vi "Motor controller.vi"   [LabVIEW 2012]
uses:
  Motors Values.vi
  BotStatus.vi
types:
  T1 = typedef "WPI_ServoDeviceRef.ctl" = cluster{"DeviceStatus":errorcluster, "Digital Module":T2, "PWM Channel":T3, "DeadBand":T4}
  T2 = typedef "FPGA_TypedefDigitalModule.ctl" = enum16{"Digital Module 1", "Digital Module 2"}
  T3 = typedef "FPGA_DIOPWMChannel.ctl" = enum8{"PWM 1", "PWM 2", "PWM 3", "PWM 4", "PWM 5", "PWM 6", "PWM 7", "PWM 8", "PWM 9", "PWM 10", "Invalid"}
  T4 = typedef "WPI_PWMDeadband.ctl" = cluster{"Name":string, "maxPositivePwm":i32, "minPositivePwm":i32, "centerPwm":i32, "maxNegativePwm":i32, "minNegativePwm":i32, "angularRange":u16}
  T5 = typedef "WPI_MotorControlDeviceRef.ctl" = cluster{"DeviceStatus":errorcluster, "Type":enum16{"PWM", "CAN"}, "PWM":cluster{"Digital Module":T2, "PWM Channel":T3, "DeadBand":T4}, "CAN":cluster{"Device Number":u8, "Control Mode":T6, "Semaphore":T7, "Max Vout":dbl}, "Invert":bool, "TransformRef":T8, "InvTransformRef":T8}
  T6 = typedef "WPI_CANJaguar_ControlMode.ctl" = enum8{"Percent VBus", "Current", "Speed", "Position", "Voltage"}
  T7 = typedef "Semaphore RefNum" = refnum<k1>
  T8 = typedef "WPI_PWMTransform_ConPane.ctl" = refnum<vi>
  T9 = typedef "WPI_RelayDevRef.ctl" = cluster{"DevStatus":errorcluster, "Relay Channel":T10, "Digital Module":T2, "Relay Direction":T11}
  T10 = typedef "FPGA_DIORelayChannel.ctl" = enum8{"Relay 1", "Relay 2", "Relay 3", "Relay 4", "Relay 5", "Relay 6", "Relay 7", "Relay 8", "Invalid"}
  T11 = typedef "WPI_RelayDirection.ctl" = enum16{"Both directions", "Forward only", "Reverse only"}
  T12 = typedef "WPI_RelayValue.ctl" = enum16{"Off", "On", "Forward", "Reverse"}
  T13 = typedef "WPI_DigitalInputDevRef.ctl" = cluster{"DevStatus":errorcluster, "DIO Channel":T14, "Digital Module":T2}
  T14 = typedef "FPGA_DIOChannel.ctl" = enum8{"DIO 1", "DIO 2", "DIO 3", "DIO 4", "DIO 5", "DIO 6", "DIO 7", "DIO 8", "DIO 9", "DIO 10", "DIO 11", "DIO 12", "DIO 13", "DIO 14", "Invalid"}
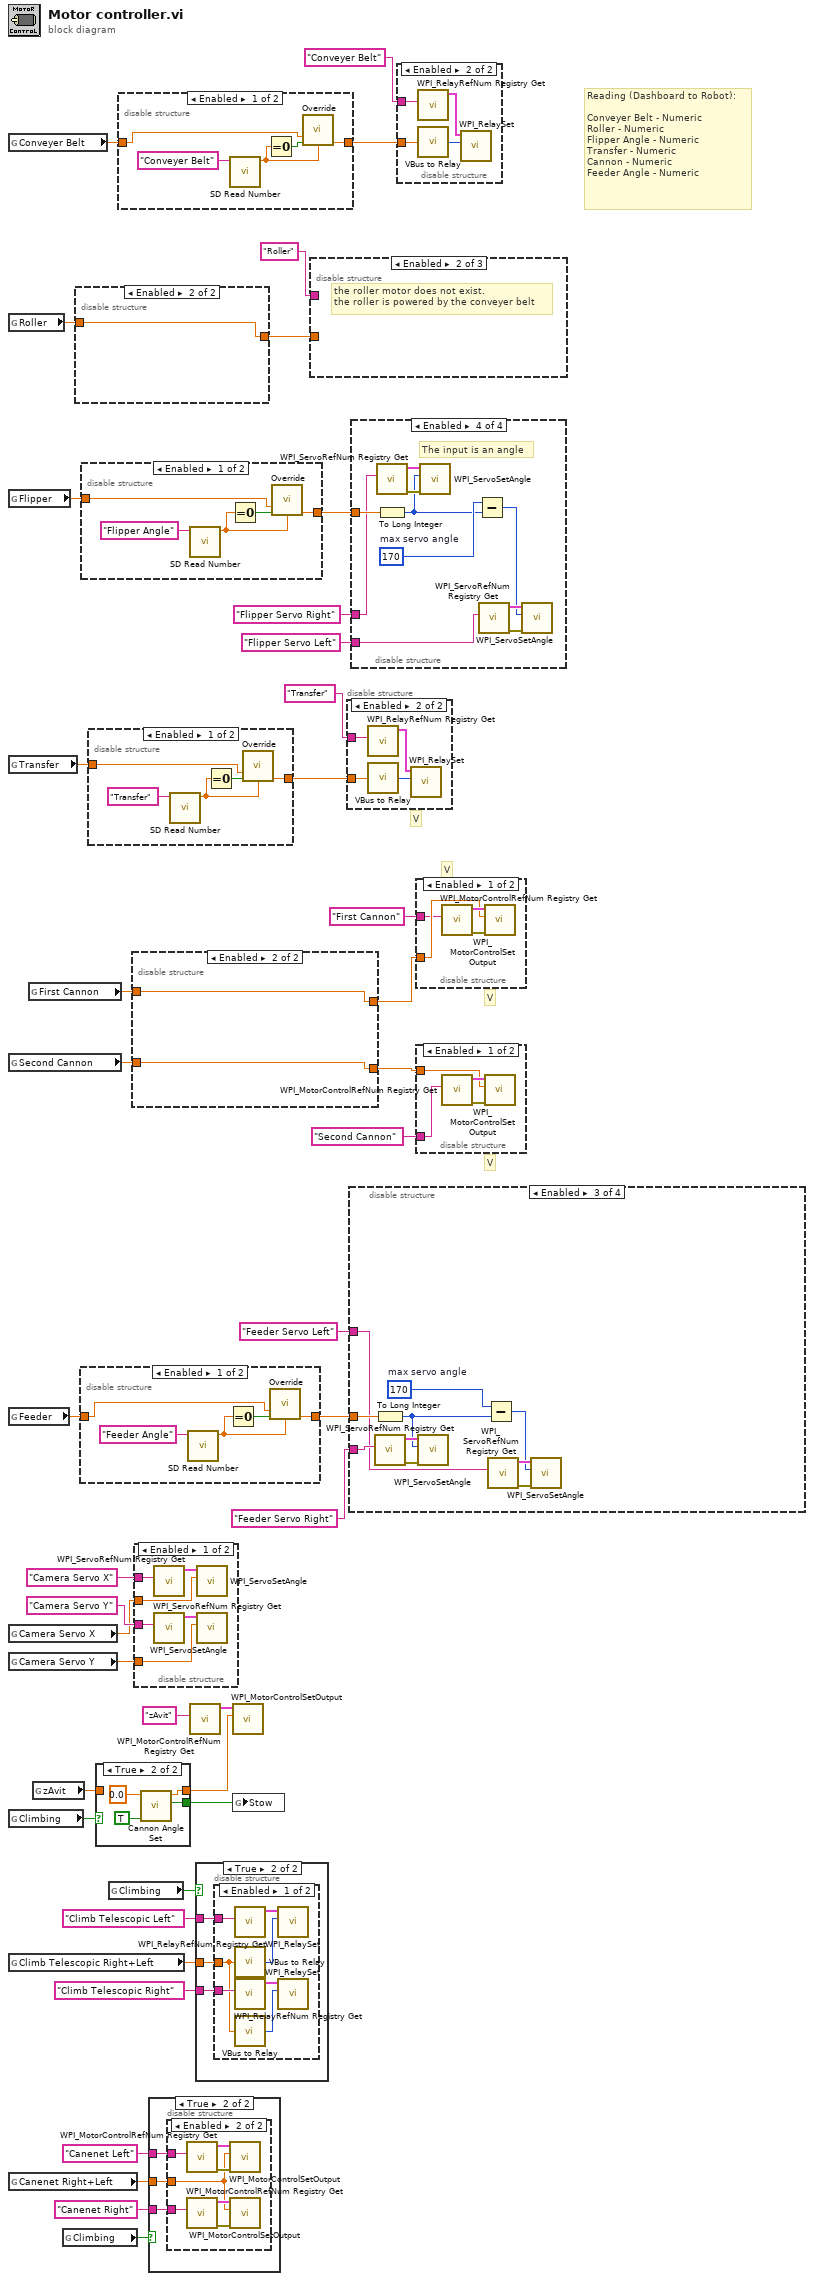
[diagram p0: block diagram]
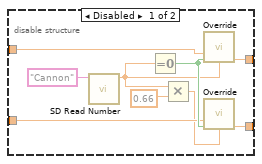
[diagram p3: hidden frame]
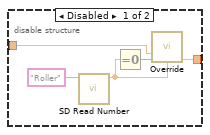
[diagram p6: hidden frame]
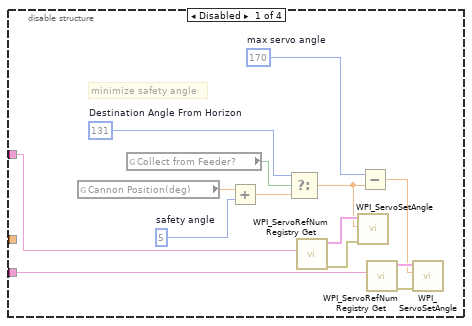
[diagram p9: hidden frame]
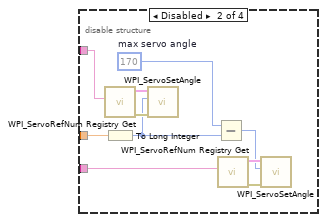
[diagram p10: hidden frame]
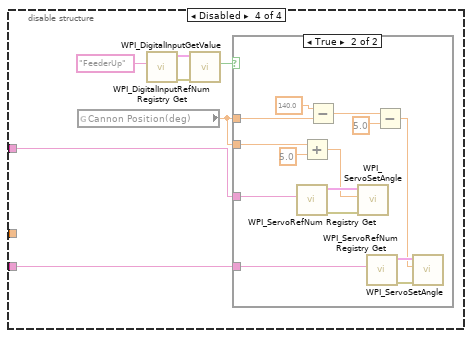
[diagram p11: hidden frame]
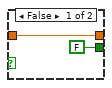
[diagram p13: hidden frame]
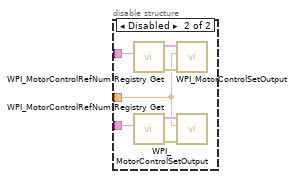
[diagram p17: hidden frame]
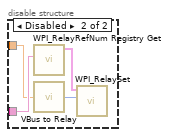
[diagram p18: hidden frame]
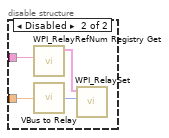
[diagram p19: hidden frame]
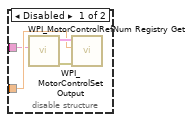
[diagram p20: hidden frame]
diagram:
  # "Reading (Dashboard to Robot):\n\nConveyer Belt - Numeric\nRoller - Numeric\nFlipper Angle - Numeric\nTransfer - Numeric\nCannon - Numeric\nFeeder Angle - Numeric"
  # "V"
  # "V"
  # "V"
  # "V"
  n1 = global read "Motors Values.vi" "Conveyer Belt"() -> (w13:dbl)
  n2 = global read "Motors Values.vi" "Roller"() -> (w12:dbl)
  n3 = global read "Motors Values.vi" "Flipper"() -> (w10:dbl)
  n4 = global read "Motors Values.vi" "Transfer"() -> (w8:dbl)
  n5 = global read "Motors Values.vi" "Second Cannon"() -> (w4:dbl)
  n6 = global read "Motors Values.vi" "Feeder"() -> (w1:dbl)
  n7 = global read "Motors Values.vi" "Camera Servo X"() -> (w16:dbl)
  n8 = global read "Motors Values.vi" "Camera Servo Y"() -> (w15:dbl)
  n9 = global read "BotStatus.vi" "Climbing"() -> (w25:bool)
  n10 = global read "Motors Values.vi" "Climb Telescopic Right+Left"() -> (w33:dbl)
  n11 = global read "Motors Values.vi" "Canenet Right+Left"() -> (w26:dbl)
  n12 = global read "Motors Values.vi" "First Cannon"() -> (w6:dbl)
  n13 = global read "Motors Values.vi" "zAvit"() -> (w24:dbl)
  n14 = global read "BotStatus.vi" "Climbing"() -> (w27:bool)
  n15 = disable-structure shown="Enabled" {
    disable-tunnel: w12 -> [w43 w47]
    disable-tunnel: [w42 w47] -> w11
    frame Disabled {
      n16 = call <vilib>:"SD Read Number.vi"("Name"="Roller") -> ("Numeric"=w45:dbl)  [unwired: 8 in, 2 out]
      n17 = Equal To 0?(x=w45) -> (x = 0?=w46:bool)
      n18 = call "Override.vi"("Regualer"=w43, "Override"=w46, "Overriden"=w45) -> ("Output"=w42:dbl)  [unwired: 12 in]
    }
    frame Enabled {
    }
  }
  n19 = disable-structure shown="Enabled" {
    disable-tunnel: [w49 w53] -> w2
    disable-tunnel: w1 -> [w48 w53]
    frame Enabled {
      n20 = call <vilib>:"SD Read Number.vi"("Name"="Feeder Angle") -> ("Numeric"=w52:dbl)  [unwired: 8 in, 2 out]
      n21 = Equal To 0?(x=w52) -> (x = 0?=w51:bool)
      n22 = call "Override.vi"("Regualer"=w48, "Override"=w51, "Overriden"=w52) -> ("Output"=w49:dbl)  [unwired: 12 in]
    }
    frame Disabled {
    }
  }
  n23 = disable-structure shown="Enabled" {
    disable-tunnel: w10 -> [w55 w59]
    disable-tunnel: [w54 w59] -> w9
    frame Enabled {
      n24 = call <vilib>:"SD Read Number.vi"("Name"="Flipper Angle") -> ("Numeric"=w57:dbl)  [unwired: 8 in, 2 out]
      n25 = Equal To 0?(x=w57) -> (x = 0?=w56:bool)
      n26 = call "Override.vi"("Regualer"=w55, "Override"=w56, "Overriden"=w57) -> ("Output"=w54:dbl)  [unwired: 12 in]
    }
    frame Disabled {
    }
  }
  n27 = disable-structure shown="Enabled" {
    disable-tunnel: w8 -> [w61 w65]
    disable-tunnel: [w60 w65] -> w7
    frame Enabled {
      n28 = call <vilib>:"SD Read Number.vi"("Name"="Transfer") -> ("Numeric"=w63:dbl)  [unwired: 8 in, 2 out]
      n29 = Equal To 0?(x=w63) -> (x = 0?=w62:bool)
      n30 = call "Override.vi"("Regualer"=w61, "Override"=w62, "Overriden"=w63) -> ("Output"=w60:dbl)  [unwired: 12 in]
    }
    frame Disabled {
    }
  }
  n31 = case shown="True" w25 {
    tunnel: [w67 w69] -> w23
    tunnel: w24 -> [w67 _]
    tunnel: [FALSE ("On Target") w68] -> w19
    frame False {
    }
    frame True {
      n32 = call "Cannon Angle Set.vi"("set angle 0 to be min angle"=TRUE, "Angle Set Point"=0.0) -> ("On Target"=w68:bool, "zAvit Vbus Out"=w69:dbl)  [unwired: 8 in]
    }
  }
  n33 = global read "BotStatus.vi" "Climbing"() -> (w32:bool)
  n34 = disable-structure shown="Enabled" {
    disable-tunnel: [w76 w77] -> w14
    disable-tunnel: w13 -> [w73 w77]
    frame Enabled {
      n35 = call <vilib>:"SD Read Number.vi"("Name"="Conveyer Belt") -> ("Numeric"=w74:dbl)  [unwired: 8 in, 2 out]
      n36 = Equal To 0?(x=w74) -> (x = 0?=w72:bool)
      n37 = call "Override.vi"("Regualer"=w73, "Override"=w72, "Overriden"=w74) -> ("Output"=w76:dbl)  [unwired: 12 in]
    }
    frame Disabled {
    }
  }
  n38 = disable-structure shown="Enabled" {
    disable-tunnel: w6 -> [w85 w88]
    disable-tunnel: [w84 w88] -> w5
    disable-tunnel: w4 -> [w82 w87]
    disable-tunnel: [w78 w87] -> w3
    frame Disabled {
      n39 = call <vilib>:"SD Read Number.vi"("Name"="Cannon") -> ("Numeric"=w81:dbl)  [unwired: 8 in, 2 out]
      n40 = Equal To 0?(x=w81) -> (x = 0?=w83:bool)
      n41 = Multiply(x=w81, y=0.66) -> (x*y=w80:dbl)
      n42 = call "Override.vi"("Regualer"=w85, "Override"=w83, "Overriden"=w81) -> ("Output"=w84:dbl)  [unwired: 12 in]
      n43 = call "Override.vi"("Regualer"=w82, "Override"=w83, "Overriden"=w80) -> ("Output"=w78:dbl)  [unwired: 12 in]
    }
    frame Enabled {
    }
  }
  n44 = disable-structure shown="Enabled" {
    disable-tunnel: "Camera Servo X" ("refnum name") -> [w93 _]
    disable-tunnel: "Camera Servo Y" ("refnum name") -> [w92 _]
    disable-tunnel: w16 -> [w90 _]
    disable-tunnel: w15 -> [w89 _]
    frame Enabled {
      n45 = call <vilib>:"WPI_ServoRefNum Registry Get.vi"("refnum name"=w93) -> ("ServoDeviceRef"=w94:T1)  [unwired: 9 in, 1 out]
      n46 = call <vilib>:"WPI_ServoRefNum Registry Get.vi"("refnum name"=w92) -> ("ServoDeviceRef"=w91:T1)  [unwired: 9 in, 1 out]
      n47 = call <vilib>:"WPI_ServoSetAngle.vi"("Angle"=w90, "ServoDeviceRef"=w94) -> ()  [unwired: 8 in, 2 out]
      n48 = call <vilib>:"WPI_ServoSetAngle.vi"("Angle"=w89, "ServoDeviceRef"=w91) -> ()  [unwired: 8 in, 2 out]
    }
    frame Disabled {
    }
  }
  n49 = case shown="True" w27 {
    tunnel: w26 -> [_ w97]
    tunnel: "Canenet Right" ("refnum name") -> [_ w96]
    tunnel: "Canenet Left" ("refnum name") -> [_ w95]
    frame False {
    }
    frame True {
      n50 = disable-structure shown="Enabled" {
        disable-tunnel: w97 -> [_ w98]
        disable-tunnel: w96 -> [_ w100]
        disable-tunnel: w95 -> [_ w99]
        frame Disabled {
        }
        frame Enabled {
          n51 = call <vilib>:"WPI_MotorControlRefNum Registry Get.vi"("refnum name"=w99) -> ("error out"=w101:errorcluster, "MotorControlDevRef"=w102:T5)  [unwired: 9 in]
          n52 = call <vilib>:"WPI_MotorControlRefNum Registry Get.vi"("refnum name"=w100) -> ("error out"=w104:errorcluster, "MotorControlDevRef"=w103:T5)  [unwired: 9 in]
          n53 = call <vilib>:"WPI_MotorControlSetOutput.vi"("error in (no error)"=w101, "Output"=w98, "MotorControlDevRef"=w102) -> ()  [unwired: 6 in, 3 out]
          n54 = call <vilib>:"WPI_MotorControlSetOutput.vi"("error in (no error)"=w104, "Output"=w98, "MotorControlDevRef"=w103) -> ()  [unwired: 6 in, 3 out]
        }
      }
    }
  }
  n55 = call <vilib>:"WPI_MotorControlRefNum Registry Get.vi"("refnum name"="zAvit") -> ("MotorControlDevRef"=w21:T5)  [unwired: 9 in, 1 out]
  n56 = case shown="True" w32 {
    tunnel: w33 -> [_ w107]
    tunnel: "Climb Telescopic Right" ("refnum name") -> [_ w106]
    tunnel: "Climb Telescopic Left" ("refnum name") -> [_ w105]
    frame False {
    }
    frame True {
      n57 = disable-structure shown="Enabled" {
        disable-tunnel: w107 -> [w109 w115]
        disable-tunnel: w106 -> [w110 w117]
        disable-tunnel: w105 -> [w111 w116]
        frame Enabled {
          n58 = call <vilib>:"WPI_RelayRefNum Registry Get.vi"("refnum name"=w111) -> ("RelayDevRef"=w113:T9)  [unwired: 9 in, 1 out]
          n59 = call "VBus to Relay.vi"("Motor VBus"=w109) -> ("RelayValue"=w112:T12)  [unwired: 3 in]
          n60 = call <vilib>:"WPI_RelayRefNum Registry Get.vi"("refnum name"=w110) -> ("RelayDevRef"=w108:T9)  [unwired: 9 in, 1 out]
          n61 = call "VBus to Relay.vi"("Motor VBus"=w109) -> ("RelayValue"=w114:T12)  [unwired: 3 in]
          n62 = call <vilib>:"WPI_RelaySet.vi"("RelayValue"=w112, "RelayDevRef"=w113) -> ()  [unwired: 8 in, 2 out]
          n63 = call <vilib>:"WPI_RelaySet.vi"("RelayValue"=w114, "RelayDevRef"=w108) -> ()  [unwired: 8 in, 2 out]
        }
        frame Disabled {
          n64 = call <vilib>:"WPI_MotorControlRefNum Registry Get.vi"("refnum name"=w116) -> ("error out"=w118:errorcluster, "MotorControlDevRef"=w119:T5)  [unwired: 9 in]
          n65 = call <vilib>:"WPI_MotorControlRefNum Registry Get.vi"("refnum name"=w117) -> ("error out"=w121:errorcluster, "MotorControlDevRef"=w120:T5)  [unwired: 9 in]
          n66 = call <vilib>:"WPI_MotorControlSetOutput.vi"("error in (no error)"=w118, "Output"=w115, "MotorControlDevRef"=w119) -> ()  [unwired: 6 in, 3 out]
          n67 = call <vilib>:"WPI_MotorControlSetOutput.vi"("error in (no error)"=w121, "Output"=w115, "MotorControlDevRef"=w120) -> ()  [unwired: 6 in, 3 out]
        }
      }
    }
  }
  n68 = call <vilib>:"WPI_MotorControlSetOutput.vi"("Output"=w23, "MotorControlDevRef"=w21) -> ()  [unwired: 7 in, 3 out]
  n69 = global write "BotStatus.vi" "Stow"(w19) -> ()
  n70 = disable-structure shown="Enabled" {
    disable-tunnel: w11 -> [w123 _ w126]
    disable-tunnel: "Roller" ("refnum name") -> [w122 _ w128]
    frame Disabled {
      n71 = call <vilib>:"WPI_MotorControlRefNum Registry Get.vi"("refnum name"=w122) -> ("error out"=w125:errorcluster, "MotorControlDevRef"=w124:T5)  [unwired: 9 in]
      n72 = call <vilib>:"WPI_MotorControlSetOutput.vi"("error in (no error)"=w125, "Output"=w123, "MotorControlDevRef"=w124) -> ()  [unwired: 6 in, 3 out]
    }
    frame Enabled {
      # "the roller motor does not exist.\nthe roller is powered by the conveyer belt"
    }
    frame Disabled {
      n73 = call <vilib>:"WPI_RelayRefNum Registry Get.vi"("refnum name"=w128) -> ("RelayDevRef"=w127:T9)  [unwired: 9 in, 1 out]
      n74 = call "VBus to Relay.vi"("Motor VBus"=w126) -> ("RelayValue"=w129:T12)  [unwired: 3 in]
      n75 = call <vilib>:"WPI_RelaySet.vi"("RelayValue"=w129, "RelayDevRef"=w127) -> ()  [unwired: 8 in, 2 out]
    }
  }
  n76 = disable-structure shown="Enabled" {
    disable-tunnel: w7 -> [w131 w134]
    disable-tunnel: "Transfer" ("refnum name") -> [w130 w136]
    frame Disabled {
      n77 = call <vilib>:"WPI_MotorControlRefNum Registry Get.vi"("refnum name"=w130) -> ("error out"=w133:errorcluster, "MotorControlDevRef"=w132:T5)  [unwired: 9 in]
      n78 = call <vilib>:"WPI_MotorControlSetOutput.vi"("error in (no error)"=w133, "Output"=w131, "MotorControlDevRef"=w132) -> ()  [unwired: 6 in, 3 out]
    }
    frame Enabled {
      n79 = call <vilib>:"WPI_RelayRefNum Registry Get.vi"("refnum name"=w136) -> ("RelayDevRef"=w135:T9)  [unwired: 9 in, 1 out]
      n80 = call "VBus to Relay.vi"("Motor VBus"=w134) -> ("RelayValue"=w137:T12)  [unwired: 3 in]
      n81 = call <vilib>:"WPI_RelaySet.vi"("RelayValue"=w137, "RelayDevRef"=w135) -> ()  [unwired: 8 in, 2 out]
    }
  }
  n82 = disable-structure shown="Enabled" {
    disable-tunnel: "Feeder Servo Left" ("refnum name") -> [w148 w153 w162 w174]
    disable-tunnel: "Feeder Servo Right" ("refnum name") -> [w145 w152 w163 w173]
    disable-tunnel: w2 -> [_ w155 w165 _]
    frame Disabled {
      w140 = 131  # Destination Angle From Horizon
      w144 = 170  # max servo angle
      w149 = 5  # safety angle
      # "minimize safety angle"
      n83 = global read "BotStatus.vi" "Cannon Position(deg)"() -> (w138:dbl)
      n84 = global read "BotStatus.vi" "Collect from Feeder?"() -> (w139:bool)
      n85 = Add(x=w138, y=w149) -> (x+y=w141:dbl)
      n86 = Select(t=w140, s=w139, f=w141) -> (s? t:f=w142:dbl)
      n87 = call <vilib>:"WPI_ServoRefNum Registry Get.vi"("refnum name"=w148) -> ("error out"=w150:errorcluster, "ServoDeviceRef"=w151:T1)  [unwired: 9 in]
      n88 = call <vilib>:"WPI_ServoSetAngle.vi"("error in (no error)"=w150, "Angle"=w142, "ServoDeviceRef"=w151) -> ()  [unwired: 7 in, 2 out]
      n89 = Subtract(x=w144, y=w142) -> (x-y=w143:dbl)
      n90 = call <vilib>:"WPI_ServoRefNum Registry Get.vi"("refnum name"=w145) -> ("error out"=w146:errorcluster, "ServoDeviceRef"=w147:T1)  [unwired: 9 in]
      n91 = call <vilib>:"WPI_ServoSetAngle.vi"("error in (no error)"=w146, "Angle"=w143, "ServoDeviceRef"=w147) -> ()  [unwired: 7 in, 2 out]
    }
    frame Disabled {
      w157 = 170  # max servo angle
      n92 = call <vilib>:"WPI_ServoRefNum Registry Get.vi"("refnum name"=w153) -> ("error out"=w160:errorcluster, "ServoDeviceRef"=w161:T1)  [unwired: 9 in]
      n93 = To Long Integer(number=w155) -> (32bit integer=w154:i32)
      n94 = call <vilib>:"WPI_ServoSetAngle.vi"("error in (no error)"=w160, "Angle"=w154, "ServoDeviceRef"=w161) -> ()  [unwired: 7 in, 2 out]
      n95 = Subtract(x=w157, y=w154) -> (x-y=w156:i32)
      n96 = call <vilib>:"WPI_ServoRefNum Registry Get.vi"("refnum name"=w152) -> ("error out"=w158:errorcluster, "ServoDeviceRef"=w159:T1)  [unwired: 9 in]
      n97 = call <vilib>:"WPI_ServoSetAngle.vi"("error in (no error)"=w158, "Angle"=w156, "ServoDeviceRef"=w159) -> ()  [unwired: 7 in, 2 out]
    }
    frame Enabled {
      w167 = 170  # max servo angle
      n98 = To Long Integer(number=w165) -> (32bit integer=w164:i32)
      n99 = call <vilib>:"WPI_ServoRefNum Registry Get.vi"("refnum name"=w163) -> ("error out"=w170:errorcluster, "ServoDeviceRef"=w171:T1)  [unwired: 9 in]
      n100 = call <vilib>:"WPI_ServoSetAngle.vi"("error in (no error)"=w170, "Angle"=w164, "ServoDeviceRef"=w171) -> ()  [unwired: 7 in, 2 out]
      n101 = Subtract(x=w167, y=w164) -> (x-y=w166:i32)
      n102 = call <vilib>:"WPI_ServoRefNum Registry Get.vi"("refnum name"=w162) -> ("error out"=w168:errorcluster, "ServoDeviceRef"=w169:T1)  [unwired: 9 in]
      n103 = call <vilib>:"WPI_ServoSetAngle.vi"("error in (no error)"=w168, "Angle"=w166, "ServoDeviceRef"=w169) -> ()  [unwired: 7 in, 2 out]
    }
    frame Disabled {
      n104 = global read "BotStatus.vi" "Cannon Position(deg)"() -> (w172:dbl)
      n105 = call <vilib>:"WPI_DigitalInputRefNum Registry Get.vi"("refnum name"="FeederUp") -> ("error out"=w176:errorcluster, "DigitalInputDevRef"=w175:T13)  [unwired: 9 in]
      n106 = call <vilib>:"WPI_DigitalInputGetValue.vi"("error in (no error)"=w176, "DigitalInputDevRef"=w175) -> ("Value"=w178:bool)  [unwired: 7 in, 2 out]
      n107 = case shown="True" w178 {
        tunnel: w174 -> [_ w190]
        tunnel: w172 -> [_ w189]
        tunnel: w173 -> [_ w181]
        tunnel: w172 -> [_ w180]
        frame False {
        }
        frame True {
          n108 = call <vilib>:"WPI_ServoRefNum Registry Get.vi"("refnum name"=w190) -> ("error out"=w191:errorcluster, "ServoDeviceRef"=w192:T1)  [unwired: 9 in]
          n109 = Add(x=w189, y=5.0) -> (x+y=w187:dbl)
          n110 = Subtract(x=140.0, y=w180) -> (x-y=w185:dbl)
          n111 = call <vilib>:"WPI_ServoSetAngle.vi"("error in (no error)"=w191, "Angle"=w187, "ServoDeviceRef"=w192) -> ()  [unwired: 7 in, 2 out]
          n112 = call <vilib>:"WPI_ServoRefNum Registry Get.vi"("refnum name"=w181) -> ("error out"=w182:errorcluster, "ServoDeviceRef"=w183:T1)  [unwired: 9 in]
          n113 = Subtract(x=w185, y=5.0) -> (x-y=w179:dbl)
          n114 = call <vilib>:"WPI_ServoSetAngle.vi"("error in (no error)"=w182, "Angle"=w179, "ServoDeviceRef"=w183) -> ()  [unwired: 7 in, 2 out]
        }
      }
    }
  }
  n115 = disable-structure shown="Enabled" {
    disable-tunnel: w9 -> [w194 w197 w207 w218]
    disable-tunnel: "Flipper Servo Left" ("refnum name") -> [w193 w199 w210 w212]
    disable-tunnel: "Flipper Servo Right" ("refnum name") -> [_ _ w201 w211]
    frame Disabled {
      n116 = call <vilib>:"WPI_MotorControlRefNum Registry Get.vi"("refnum name"=w193) -> ("error out"=w196:errorcluster, "MotorControlDevRef"=w195:T5)  [unwired: 9 in]
      n117 = call <vilib>:"WPI_MotorControlSetOutput.vi"("error in (no error)"=w196, "Output"=w194, "MotorControlDevRef"=w195) -> ()  [unwired: 6 in, 3 out]
    }
    frame Disabled {
      n118 = call <vilib>:"WPI_RelayRefNum Registry Get.vi"("refnum name"=w199) -> ("RelayDevRef"=w198:T9)  [unwired: 9 in, 1 out]
      n119 = call "VBus to Relay.vi"("Motor VBus"=w197) -> ("RelayValue"=w200:T12)  [unwired: 3 in]
      n120 = call <vilib>:"WPI_RelaySet.vi"("RelayValue"=w200, "RelayDevRef"=w198) -> ()  [unwired: 8 in, 2 out]
    }
    frame Disabled {
      w204 = 170  # max servo angle
      # "The input is an angle"
      n121 = To Long Integer(number=w207) -> (32bit integer=w203:i32)
      n122 = call <vilib>:"WPI_ServoRefNum Registry Get.vi"("refnum name"=w210) -> ("error out"=w208:errorcluster, "ServoDeviceRef"=w209:T1)  [unwired: 9 in]
      n123 = call <vilib>:"WPI_ServoSetAngle.vi"("error in (no error)"=w208, "Angle"=w203, "ServoDeviceRef"=w209) -> ()  [unwired: 7 in, 2 out]
      n124 = Subtract(x=w204, y=w203) -> (x-y=w202:i32)
      n125 = call <vilib>:"WPI_ServoRefNum Registry Get.vi"("refnum name"=w201) -> ("error out"=w206:errorcluster, "ServoDeviceRef"=w205:T1)  [unwired: 9 in]
      n126 = call <vilib>:"WPI_ServoSetAngle.vi"("error in (no error)"=w206, "Angle"=w202, "ServoDeviceRef"=w205) -> ()  [unwired: 7 in, 2 out]
    }
    frame Enabled {
      w215 = 170  # max servo angle
      # "The input is an angle"
      n127 = call <vilib>:"WPI_ServoRefNum Registry Get.vi"("refnum name"=w211) -> ("error out"=w219:errorcluster, "ServoDeviceRef"=w220:T1)  [unwired: 9 in]
      n128 = To Long Integer(number=w218) -> (32bit integer=w214:i32)
      n129 = call <vilib>:"WPI_ServoSetAngle.vi"("error in (no error)"=w219, "Angle"=w214, "ServoDeviceRef"=w220) -> ()  [unwired: 7 in, 2 out]
      n130 = Subtract(x=w215, y=w214) -> (x-y=w213:i32)
      n131 = call <vilib>:"WPI_ServoRefNum Registry Get.vi"("refnum name"=w212) -> ("error out"=w217:errorcluster, "ServoDeviceRef"=w216:T1)  [unwired: 9 in]
      n132 = call <vilib>:"WPI_ServoSetAngle.vi"("error in (no error)"=w217, "Angle"=w213, "ServoDeviceRef"=w216) -> ()  [unwired: 7 in, 2 out]
    }
  }
  n133 = disable-structure shown="Enabled" {
    disable-tunnel: w14 -> [w222 w225]
    disable-tunnel: "Conveyer Belt" ("refnum name") -> [w221 w227]
    frame Disabled {
      n134 = call <vilib>:"WPI_MotorControlRefNum Registry Get.vi"("refnum name"=w221) -> ("error out"=w224:errorcluster, "MotorControlDevRef"=w223:T5)  [unwired: 9 in]
      n135 = call <vilib>:"WPI_MotorControlSetOutput.vi"("error in (no error)"=w224, "Output"=w222, "MotorControlDevRef"=w223) -> ()  [unwired: 6 in, 3 out]
    }
    frame Enabled {
      n136 = call <vilib>:"WPI_RelayRefNum Registry Get.vi"("refnum name"=w227) -> ("RelayDevRef"=w226:T9)  [unwired: 9 in, 1 out]
      n137 = call "VBus to Relay.vi"("Motor VBus"=w225) -> ("RelayValue"=w228:T12)  [unwired: 3 in]
      n138 = call <vilib>:"WPI_RelaySet.vi"("RelayValue"=w228, "RelayDevRef"=w226) -> ()  [unwired: 8 in, 2 out]
    }
  }
  n139 = disable-structure shown="Enabled" {
    disable-tunnel: w5 -> [w230 w233]
    disable-tunnel: "First Cannon" ("refnum name") -> [w229 w235]
    frame Enabled {
      n140 = call <vilib>:"WPI_MotorControlRefNum Registry Get.vi"("refnum name"=w229) -> ("error out"=w232:errorcluster, "MotorControlDevRef"=w231:T5)  [unwired: 9 in]
      n141 = call <vilib>:"WPI_MotorControlSetOutput.vi"("error in (no error)"=w232, "Output"=w230, "MotorControlDevRef"=w231) -> ()  [unwired: 6 in, 3 out]
    }
    frame Disabled {
      n142 = call <vilib>:"WPI_RelayRefNum Registry Get.vi"("refnum name"=w235) -> ("RelayDevRef"=w234:T9)  [unwired: 9 in, 1 out]
      n143 = call "VBus to Relay.vi"("Motor VBus"=w233) -> ("RelayValue"=w236:T12)  [unwired: 3 in]
      n144 = call <vilib>:"WPI_RelaySet.vi"("RelayValue"=w236, "RelayDevRef"=w234) -> ()  [unwired: 8 in, 2 out]
    }
  }
  n145 = disable-structure shown="Enabled" {
    disable-tunnel: w3 -> [w238 w241]
    disable-tunnel: "Second Cannon" ("refnum name") -> [w237 w243]
    frame Enabled {
      n146 = call <vilib>:"WPI_MotorControlRefNum Registry Get.vi"("refnum name"=w237) -> ("error out"=w240:errorcluster, "MotorControlDevRef"=w239:T5)  [unwired: 9 in]
      n147 = call <vilib>:"WPI_MotorControlSetOutput.vi"("error in (no error)"=w240, "Output"=w238, "MotorControlDevRef"=w239) -> ()  [unwired: 6 in, 3 out]
    }
    frame Disabled {
      n148 = call <vilib>:"WPI_RelayRefNum Registry Get.vi"("refnum name"=w243) -> ("RelayDevRef"=w242:T9)  [unwired: 9 in, 1 out]
      n149 = call "VBus to Relay.vi"("Motor VBus"=w241) -> ("RelayValue"=w244:T12)  [unwired: 3 in]
      n150 = call <vilib>:"WPI_RelaySet.vi"("RelayValue"=w244, "RelayDevRef"=w242) -> ()  [unwired: 8 in, 2 out]
    }
  }
